vi "Ingest Data.vi"(8 "error in":errorcluster, 10 "NewData":refnum<class "PAS Data.lvclass">, 11 "OldData":refnum<class "PAS Data.lvclass">) -> (0 "error out":errorcluster, 3 "PAS Data out":refnum<class "PAS Data.lvclass">)   [LabVIEW 2014]
doc: "Ingest data while maintaining the reference to the binary file."
uses:
  PAS Data.lvclass
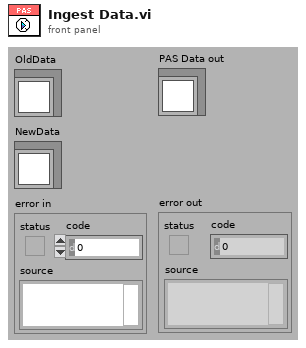
[diagram p1: front panel]
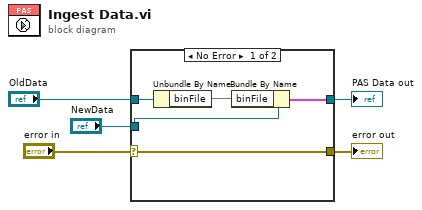
[diagram p0: block diagram]
diagram:
  n1 = case shown="No Error" "error in" {
    selector: "error in" -> [w10 w12]
    tunnel: [w10 w12] -> w4
    tunnel: [w6 w11] -> w2
    tunnel: "OldData" -> [w9 w11]
    tunnel: "NewData" -> [w8 _]
    frame No Error {
      n2 = Unbundle By Name(w9) -> ("binFile"=w7)
      n3 = Bundle By Name(cluster=w8, "binFile"=w7) -> (w6:cluster{})
    }
    frame Error {
    }
  }
  "error out" <- w4
  "PAS Data out" <- w2
